vi "Get Switch Device Names.vi"(0 "IVI Specifications":string[][](array[string]), 3 "error in (no error)":errorcluster) -> (7 "Device Names":string[](array[string]), 10 "error out":errorcluster)   [LabVIEW 2019]
uses:
  be71f759-0074-4cad-bee4-44019e47bee5.vi
  77d57afb-d4b4-4974-ac3b-3e792e1df93a.vi
  <instrlib>/niModInst/niModInst Get Installed Device Attribute (String).vi
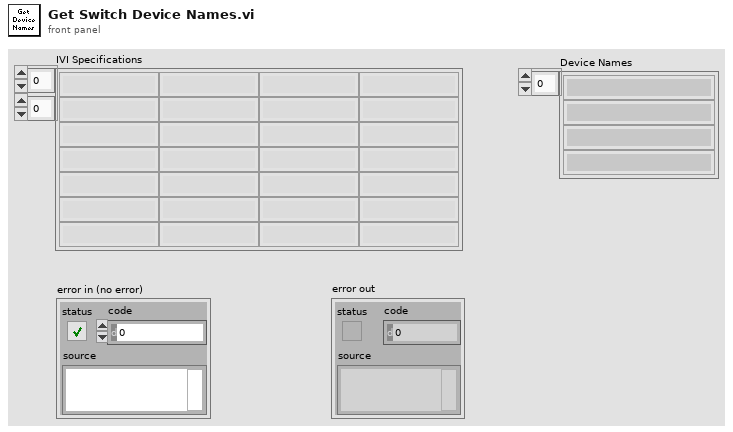
[diagram p1: front panel]
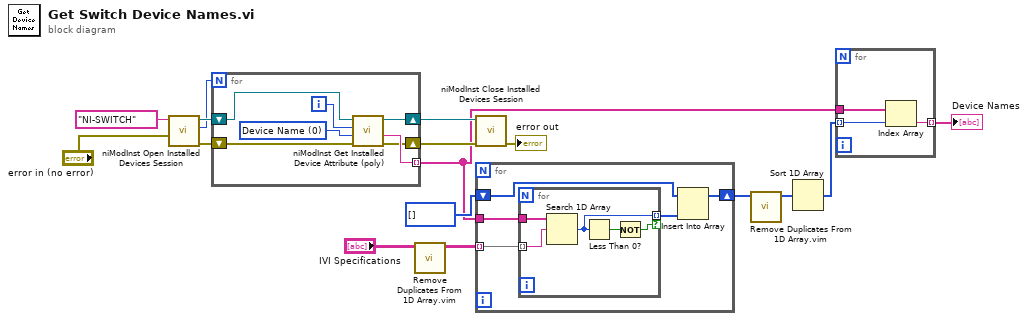
[diagram p0: block diagram]
diagram:
  n1 = call <instrlib>:"niModInst Open Installed Devices Session.vi"("error in (no error)"="error in (no error)", "driver"="NI-SWITCH") -> ("error out"=w14:errorcluster, "device count"=w13:i32, "session"=w15:refnum<k20>)  [unwired: 7 in]
  n2 = for {
    N: w13 -> [_]
    tunnel: [w19] -> w7 mode=indexing
    shift-right: [w18] -> w12
    shift-left: w15 -> [w23]
    shift-right: [w17] -> w11
    shift-left: w14 -> [w22]
    i -> [w21]
    w20 = 0 items=["Device Name", "Device Model", "Serial Number"] ("attribute ID")
    n3 = call-poly <instrlib>:"niModInst Get Installed Device Attribute (poly).vi"("error in (no error)"=w22, "attribute ID"=w20, "index in"=w21, "session in"=w23) -> ("error out"=w17:errorcluster, "attribute value"=w19:string, "session out"=w18:refnum<k20>)  [unwired: 4 in, 1 out]
  }
  n4 = call "Remove Duplicates From 1D Array.vim"("array"="IVI Specifications") -> ("array with duplicates removed"=w4:string[][])  [unwired: 10 in]
  n5 = call <instrlib>:"niModInst Close Installed Devices Session.vi"("error in (no error)"=w11, "session"=w12) -> ("error out"=→"error out":errorcluster)  [unwired: 9 in]
  n6 = for {
    tunnel: w4 -> [w28] mode=indexing
    tunnel: w7 -> [w27]
    shift-right: [w24] -> w9
    shift-left: i32[] [] -> [w25]
    n7 = for {
      tunnel: w28 -> [w33] mode=indexing
      tunnel: w27 -> [w32]
      tunnel: [w31] -> w26 mode=indexing if=w29
      n8 = Search 1D Array(1D array=w32, element=w33) -> (index of element=w31:i32)  [unwired: 1 in]
      n9 = Less Than 0?(x=w31) -> (x < 0?=w30:bool)
      n10 = Not(x=w30) -> (.not. x?=w29:bool)
    }
    n11 = Insert Into Array(array=w25, new element=w26) -> (w24:i32[])  [unwired: 1 in]
  }
  n12 = call "Remove Duplicates From 1D Array.vim"("array"=w9) -> ("array with duplicates removed"=w8:i32[])  [unwired: 10 in]
  n13 = Sort 1D Array(array=w8) -> (sorted array=w6:i32[])
  n14 = for {
    tunnel: w7 -> [w36]
    tunnel: w6 -> [w35] mode=indexing
    tunnel: [w34] -> w5 mode=indexing
    n15 = Index Array(array=w36, index=w35) -> (element=w34:string)
  }
  "Device Names" <- w5
